vi "get_sample_delay.vi"(8 "error in (no error)":errorcluster, 11 "GenericWriteSignals in":refnum<class "GenericSignalWriter.lvclass">) -> (0 "error out":errorcluster, 2 "sample delay (samples)":i32, 3 "GenericWriteSignals out":refnum<class "GenericSignalWriter.lvclass">)   [LabVIEW 2010, in "GenericSignalWriter.lvclass"]
uses:
  GenericSignalWriter.lvclass
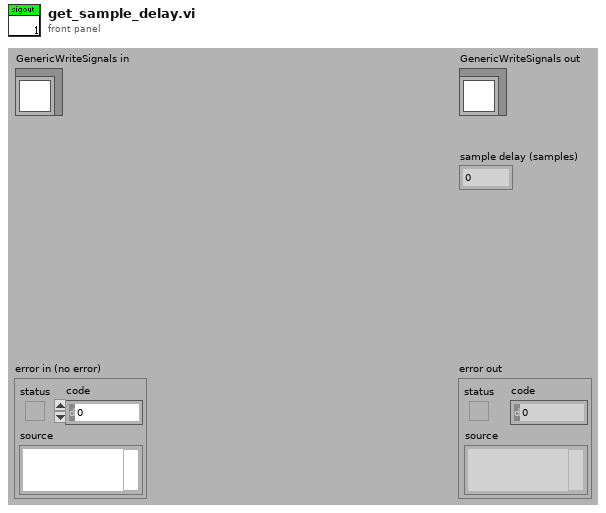
[diagram p1: front panel]
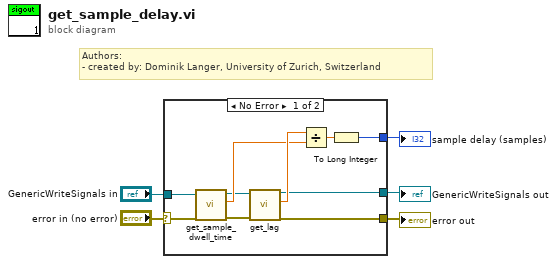
[diagram p0: block diagram]
diagram:
  # "Authors: \n- created by: Dominik Langer, University of Zurich, Switzerland"
  n1 = case shown="No Error" "error in (no error)" {
    selector: "error in (no error)" -> [w8 w17]
    tunnel: [w7 w17] -> w4
    tunnel: [w9 w16] -> w2
    tunnel: "GenericWriteSignals in" -> [w10 w16]
    tunnel: [w6 _] -> w1
    frame No Error {
      n2 = call-dynamic "get_sample_dwell_time.vi"("error in (no error)"=w8, "GenericWriteSignals.lvclass in"=w10) -> ("error out"=w14:errorcluster, "sample dwell time"=w13:dbl[unit], "GenericWriteSignals.lvclass out"=w11:refnum<class "GenericSignalWriter.lvclass">)  [unwired: 7 out]
      n3 = call-dynamic "get_lag.vi"("error in (no error)"=w14, "GenericWriteSignals.lvclass in"=w11) -> ("error out"=w7:errorcluster, "lag"=w15:dbl[unit], "GenericWriteSignals.lvclass out"=w9:refnum<class "GenericSignalWriter.lvclass">)  [unwired: 7 out]
      n4 = Divide(x=w15, y=w13) -> (x/y=w12:dbl)
      n5 = To Long Integer(number=w12) -> (32bit integer=w6:i32)
    }
    frame Error {
    }
  }
  "error out" <- w4
  "GenericWriteSignals out" <- w2
  "sample delay (samples)" <- w1
